vi "keithleyCount.vi"(11 "Action":enum16{"Read", "increment", "deincrement"}(ring)) -> (2 "Numeric":i32)   [LabVIEW 2011, in "Hardware.lvlib" / "Channels.lvlib"]
uses:
  Channels.lvlib
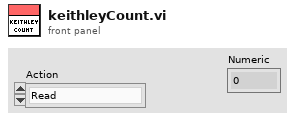
[diagram p1: front panel]
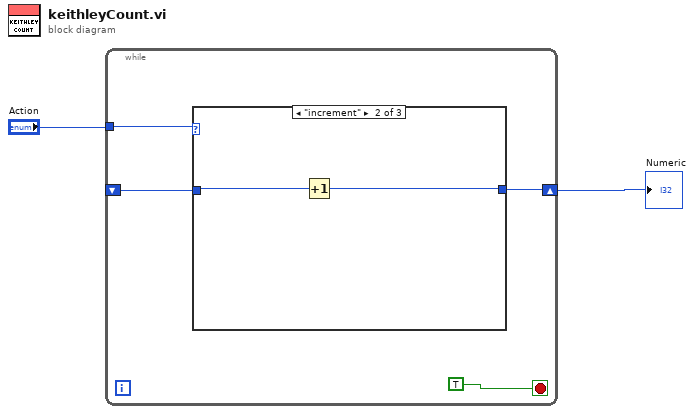
[diagram p0: block diagram]
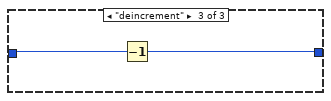
[diagram p3: hidden frame]
diagram:
  n1 = while {
    tunnel: "Action" -> [w6]
    shift-right: [w4] -> w1
    shift-left: _ -> [w3]
    stop <- TRUE stop-if-true
    n2 = case shown="\"increment\"" w6 {
      tunnel: [w7 w8 w10] -> w4
      tunnel: w3 -> [w7 w9 w11]
      frame "Read", Default {
      }
      frame "increment" {
        n3 = Increment(x=w9) -> (x+1=w8:i32)
      }
      frame "deincrement" {
        n4 = Decrement(x=w11) -> (x-1=w10:i32)
      }
    }
  }
  "Numeric" <- w1
